vi "WSVCAP SHL FPGA LL Procedure I2C - Send Start or Stop Sequence.vi"(0 "Procedure Step":T1, 1 "Wait Ticks Remaining":u32, 5 "I2C Wait Ticks":u32, 11 "error in (no error)":errorcluster, 12 "Type (T:Start; F:Stop)":bool, 13 "Socket Mask":u64, 14 "UUT Set (0/1)":u8) -> (3 "Wait Ticks Remaining Out":u32, 4 "Procedure Step Out":T1, 8 "Finished":bool, 15 "error out":errorcluster)   [LabVIEW 2017]
uses:
  Type Defs/WSVCAP SHL Procedure Step Enum.ctl
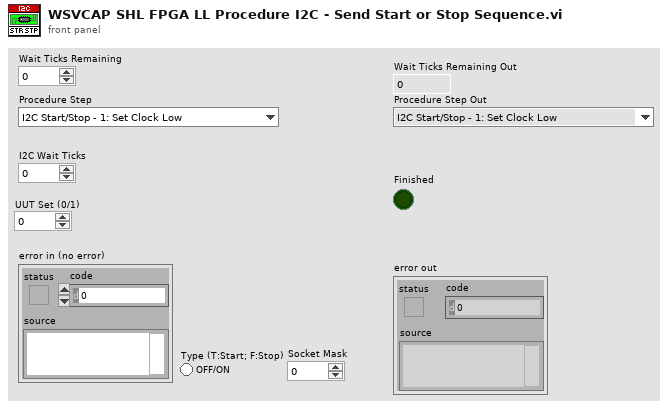
[diagram p1: front panel]
types:
  T1 = typedef "WSVCAP SHL Procedure Step Enum.ctl" = enum16{"I2C Start/Stop - 1: Set Clock Low", "I2C Start/Stop - 2: Wait", "I2C Start/Stop - 3: Set Data I", "I2C Start/Stop - 4: Wait", "I2C Start/Stop - 5: Set Clock High", "I2C Start/Stop - 6: Wait", "I2C Start/Stop - 7: Set Data II", "I2C Start/Stop - 8: Wait", "I2C Start/Stop - 9: Set Clock Low", "I2C Start/Stop - 10: Wait", "I2C Read ACK - 1: Set Clock High", "I2C Read ACK - 2: Wait", "I2C Read ACK - 3: Read ACK Bit", "I2C Read ACK - 4: Wait", "I2C Read ACK - 5: Set Clock Low", "I2C Read ACK - 6: Wait", "I2C Write ACK - 1: Write ACK Bit", "I2C Write ACK - 2: Wait", "I2C Write ACK - 3: Set Clock High", "I2C Write ACK - 4: Wait", "I2C Write ACK - 5: Set Clock Low", "I2C Write ACK - 6: Wait", "I2C Write ACK - 7: Set Data Low", "I2C Send Add - 1: Reset Bits Remaining", "I2C Send Add - 2: Set Data Bit", "I2C Send Add - 3: Wait", "I2C Send Add - 4: Set Clock High", "I2C Send Add - 5: Wait", "I2C Send Add - 6: Set Clock Low", "I2C Send Add - 7: Wait", "I2C Send Add - 8: Check Bits Remaining", "I2C Send Data - 1: Reset Bits Remaining", "I2C Send Data - 2: Load Write Bit from FIFO", "I2C Send Data - 3: Set Data Bit", "I2C Send Data - 4: Wait", "I2C Send Data - 5: Set Clock High", "I2C Send Data - 6: Wait", "I2C Send Data - 7: Set Clock Low", "I2C Send Data - 8: Wait", "I2C Send Data - 9: Check Bits Remaining", "I2C Receive Data - 1: Reset Bits Remaining", "I2C Receive Data - 2: Wait", "I2C Receive Data - 3: Set Clock High", "I2C Receive Data - 4: Wait", "I2C Receive Data - 5: Read Data Bit", "I2C Receive Data - 6: Wait", "I2C Receive Data - 7: Set Clock Low", "I2C Receive Data - 8: Wait", "I2C Receive Data - 9: Check Bits Remaining", "RFFE Send SSC - 1:Set Low", "RFFE Send SSC - 2:Wait", "RFFE Send SSC - 3:Set SDA High", "RFFE Send SSC - 4:Wait", "RFFE Send SSC - 5:Set SDA Low", "RFFE Send SSC - 6:Wait", "RFFE Send Data - 1:Set SCL High", "RFFE Send Data - 2:Wait", "RFFE Send Data - 3:Set SCL Low", "RFFE Send Data - 4:Wait", "RFFE Send Data - 5:Set SCL High (P)", "RFFE Send Data - 6:Wait", "RFFE Send Data - 7:Set SCL Low (P)", "RFFE Send Data - 8:Wait", "RFFE Send Data - 9:Set SCL High (BP)", "RFFE Send Data - 10:Wait", "RFFE Send Data - 11:Set SCL Low (BP)", "RFFE Send Data - 12:Wait", "RFFE Receive Data - 1:Set SCL High", "RFFE Receive Data - 2:Wait", "RFFE Receive Data - 3:Set SCL Low", "RFFE Receive Data - 4:Wait", "RFFE Receive Data - 5:Set SCL High (BP)", "RFFE Receive Data - 6:Wait", "RFFE Receive Data - 7:Set SCL Low (BP)", "RFFE Receive Data - 8:Wait", "RFFE Wait CMD Delay - 1:Wait", "RFFE Clear Lines - 1:Clear"}
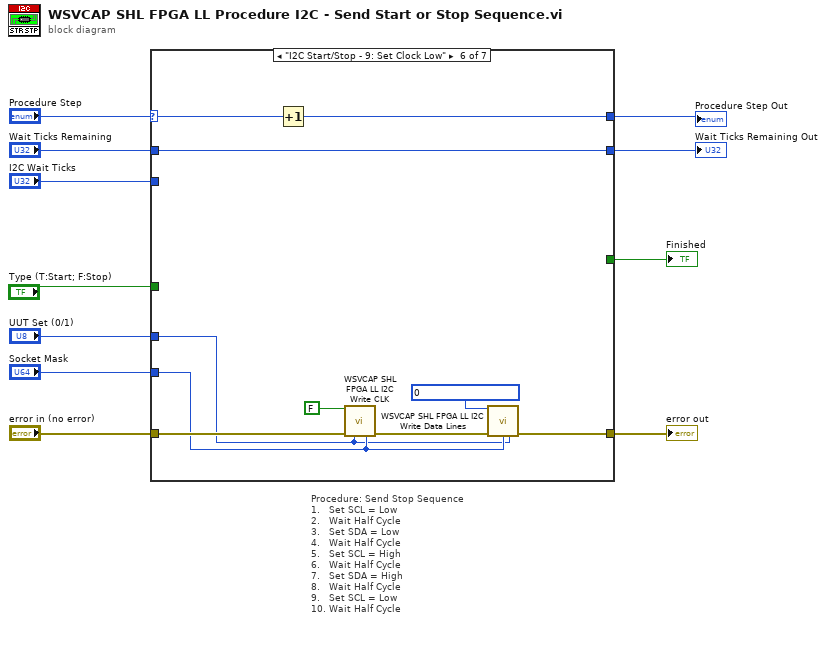
[diagram p0: block diagram]
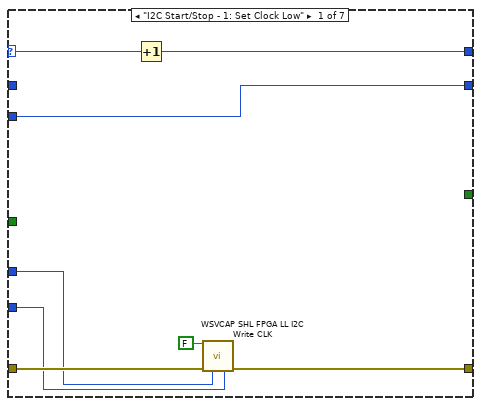
[diagram p2: hidden frame]
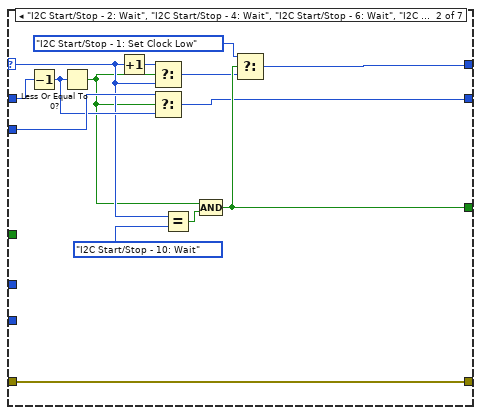
[diagram p3: hidden frame]
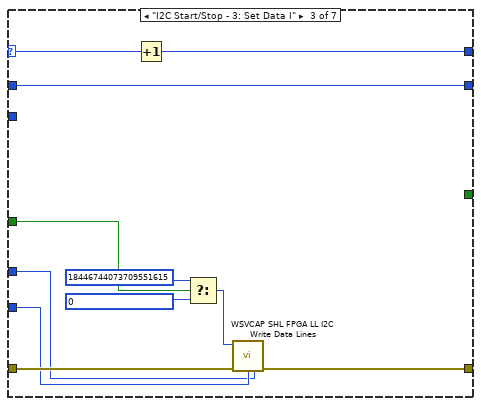
[diagram p4: hidden frame]
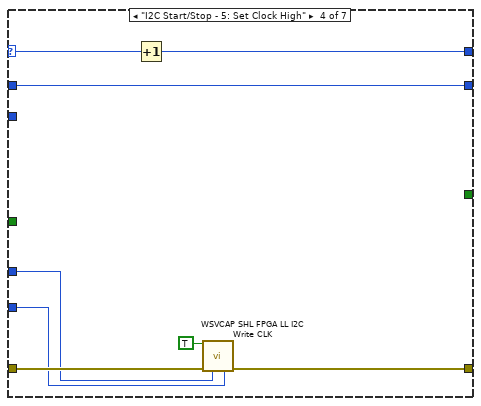
[diagram p5: hidden frame]
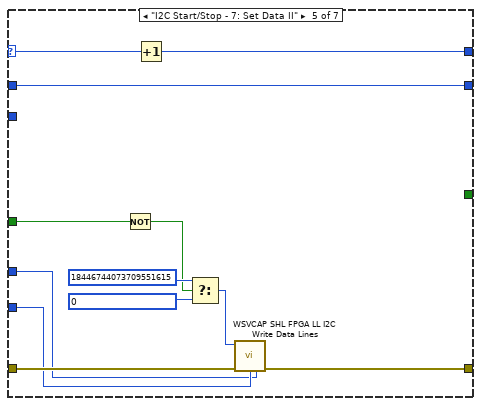
[diagram p6: hidden frame]
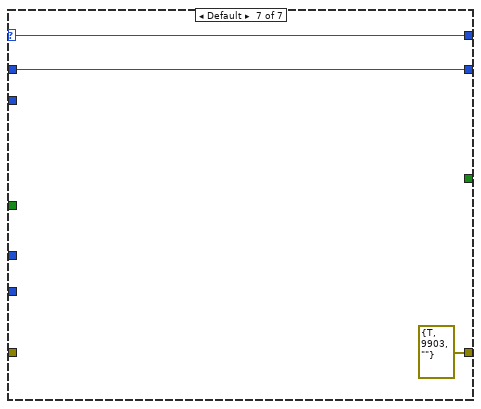
[diagram p7: hidden frame]
diagram:
  # "Procedure: Send Stop Sequence\n1.   Set SCL = Low\n2.   Wait Half Cycle\n3.   Set SDA = Low\n4.   Wait Half Cycle\n5.   Set SCL = High\n6.   Wait Half Cycle\n7.   Set SDA = High\n8.   Wait Half Cycle\n9.   Set SCL = Low\n10. Wait Half Cycle"
  n1 = case shown="\"I2C Start/Stop - 9: Set Clock Low\"" "Procedure Step" {
    selector: "Procedure Step" -> [w16 w28 w44 w49 w64 w72 w76]
    tunnel: [w18 w31 w36 w51 w56 w68 errorcluster {"status"=TRUE, "code"=9903, "source"=""} ("error out")] -> w10
    tunnel: "error in (no error)" -> [w19 w31 w37 w52 w57 w74 _]
    tunnel: "Wait Ticks Remaining" -> [_ w33 w42 w46 w61 w70 w75]
    tunnel: "I2C Wait Ticks" -> [w13 w30 _ _ _ _ _]
    tunnel: [_ w25 _ _ _ _ _] -> w9
    tunnel: "Socket Mask" -> [w15 _ w35 w48 w55 w66 _]
    tunnel: "Type (T:Start; F:Stop)" -> [_ _ w38 _ w63 _ _]
    tunnel: [w14 w21 w43 w47 w62 w71 w76] -> w3
    tunnel: [w13 w20 w42 w46 w61 w70 w75] -> w2
    tunnel: "UUT Set (0/1)" -> [w12 _ w34 w45 w54 w65 _]
    frame "I2C Start/Stop - 1: Set Clock Low" {
      n2 = Increment(x=w16) -> (x+1=w14:T1)
      n3 = call "WSVCAP SHL FPGA LL I2C Write CLK.vi"("Bit In"=FALSE, "error in (no error)"=w19, "UUT Set (0/1 (Legacy)"=w12, "Socket Mask"=w15) -> ("error out"=w18:errorcluster)  [unwired: 11 in]
    }
    frame "I2C Start/Stop - 2: Wait", "I2C Start/Stop - 4: Wait", "I2C Start/Stop - 6: Wait", "I2C Start/Stop - 8: Wait", "I2C Start/Stop - 10: Wait" {
      n4 = Decrement(x=w33) -> (x-1=w29:u32)
      n5 = Less Or Equal To 0?(x=w29) -> (x <= 0?=w27:bool)
      n6 = Increment(x=w28) -> (x+1=w32:T1)
      n7 = Select(t=w32, s=w27, f=w28) -> (s? t:f=w24:T1)
      n8 = Select(t=w30, s=w27, f=w29) -> (s? t:f=w20:u32)
      n9 = Equal?(x=w28, y=WSVCAP_SHL_Procedure_Step_Enum."I2C Start/Stop - 10: Wait" ("Procedure Step")) -> (x = y?=w26:bool)
      n10 = Compound Arithmetic op=AND(w27, w26) -> (w25:bool)
      n11 = Select(t=WSVCAP_SHL_Procedure_Step_Enum."I2C Start/Stop - 1: Set Clock Low" ("Procedure Step"), s=w25, f=w24) -> (s? t:f=w21:T1)
    }
    frame "I2C Start/Stop - 3: Set Data I" {
      n12 = Increment(x=w44) -> (x+1=w43:T1)
      n13 = Select(t=u64 18446744073709551615 ("Write Bit (U64)"), s=w38, f=u64 0 ("Write Bit (U64)")) -> (s? t:f=w39:u64)
      n14 = call "WSVCAP SHL FPGA LL I2C Write Data Lines.vi"("Write Bit (U64)"=w39, "error in (no error)"=w37, "Socket Mask"=w35, "UUT Set (0/1) (Legacy)"=w34) -> ("error out"=w36:errorcluster)  [unwired: 11 in]
    }
    frame "I2C Start/Stop - 5: Set Clock High" {
      n15 = Increment(x=w49) -> (x+1=w47:T1)
      n16 = call "WSVCAP SHL FPGA LL I2C Write CLK.vi"("Bit In"=TRUE, "error in (no error)"=w52, "UUT Set (0/1 (Legacy)"=w45, "Socket Mask"=w48) -> ("error out"=w51:errorcluster)  [unwired: 11 in]
    }
    frame "I2C Start/Stop - 7: Set Data II" {
      n17 = Not(x=w63) -> (.not. x?=w53:bool)
      n18 = Increment(x=w64) -> (x+1=w62:T1)
      n19 = Select(t=u64 18446744073709551615 ("Write Bit (U64)"), s=w53, f=u64 0 ("Write Bit (U64)")) -> (s? t:f=w58:u64)
      n20 = call "WSVCAP SHL FPGA LL I2C Write Data Lines.vi"("Write Bit (U64)"=w58, "error in (no error)"=w57, "Socket Mask"=w55, "UUT Set (0/1) (Legacy)"=w54) -> ("error out"=w56:errorcluster)  [unwired: 11 in]
    }
    frame "I2C Start/Stop - 9: Set Clock Low" {
      n21 = Increment(x=w72) -> (x+1=w71:T1)
      n22 = call "WSVCAP SHL FPGA LL I2C Write CLK.vi"("Bit In"=FALSE, "error in (no error)"=w74, "UUT Set (0/1 (Legacy)"=w65, "Socket Mask"=w66) -> ("error out"=w69:errorcluster)  [unwired: 11 in]
      n23 = call "WSVCAP SHL FPGA LL I2C Write Data Lines.vi"("Write Bit (U64)"=u64 0, "error in (no error)"=w69, "Socket Mask"=w66, "UUT Set (0/1) (Legacy)"=w65) -> ("error out"=w68:errorcluster)  [unwired: 11 in]
    }
    frame Default {
    }
  }
  "error out" <- w10
  "Finished" <- w9
  "Wait Ticks Remaining Out" <- w2
  "Procedure Step Out" <- w3
